vi "Extract Scaling Info.vi"(0 "TDMS In":refnum<k34>, 11 "Error In":errorcluster) -> (4 "TDMS Out":refnum<k34>, 6 "Inputs Scaling":T1, 10 "Outputs Scaling":T1, 15 "Error Out":errorcluster)   [LabVIEW 2015, in "Teaching File.lvlib"]
doc: "Extract scaling information using the min and max arrays for IO channels in the teaching file."
uses:
  Teaching File/Teaching File.lvlib
  Types/Scaling Info.ctl
  Neural Network.lvclass
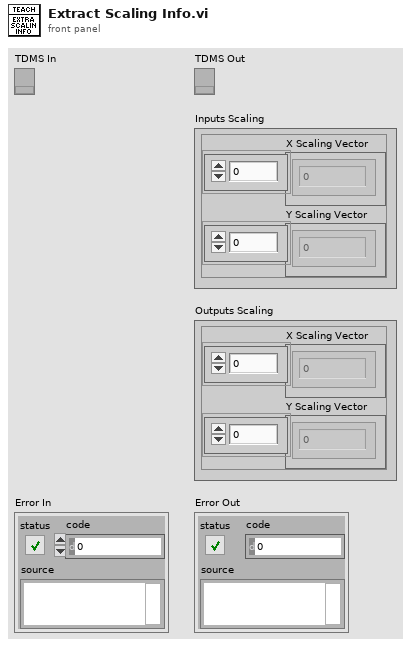
[diagram p1: front panel]
types:
  T1 = typedef "Neural Network.lvclass/Scaling Info.ctl" = cluster{"X Scaling Vector":dbl[], "Y Scaling Vector":dbl[]}
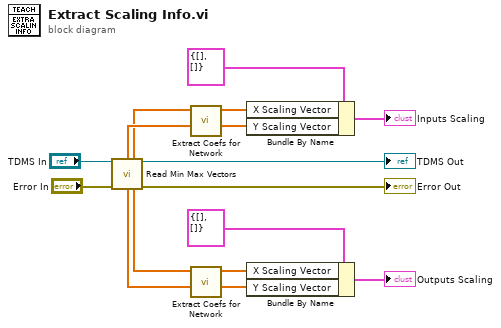
[diagram p0: block diagram]
diagram:
  n1 = call "Read Min Max Vectors.vi"("TDMS In"="TDMS In", "Error In"="Error In") -> ("Inputs Min"=w7:dbl[], "Inputs Max"=w6:dbl[], "TDMS Out"=→"TDMS Out":refnum<k34>, "Outputs Min"=w4:dbl[], "Outputs Max"=w5:dbl[], "Error Out"=→"Error Out":errorcluster)  [unwired: 8 in]
  n2 = call "Extract Coefs for Network.vi"("Min Array"=w7, "Max Array"=w6) -> ("Y Scaling Vector"=w9:dbl[], "X Scaling Vector"=w8:dbl[])  [unwired: 8 in]
  n3 = call "Extract Coefs for Network.vi"("Min Array"=w4, "Max Array"=w5) -> ("Y Scaling Vector"=w12:dbl[], "X Scaling Vector"=w11:dbl[])  [unwired: 8 in]
  n4 = Bundle By Name(cluster=T1 {"X Scaling Vector"=[], "Y Scaling Vector"=[]}, "X Scaling Vector"=w8, "Y Scaling Vector"=w9) -> (→"Inputs Scaling":T1)
  n5 = Bundle By Name(cluster=T1 {"X Scaling Vector"=[], "Y Scaling Vector"=[]}, "X Scaling Vector"=w11, "Y Scaling Vector"=w12) -> (→"Outputs Scaling":T1)
